vi "SimpleLiveApp.vi"() -> ()   [LabVIEW 2018]
uses:
  C:/Users/Public/Documents/Photometrics/PMQI-LabViewSamples/Examples/Dependencies/PVCamNET.dll
  Public/Documents/Photometrics/PMQI-LabViewSamples/Examples/Dependencies/PVCamNET.dll
panel:
  in  "Exposure Time":dbl
  in  "Live":bool
  in  "Camera Status":bool
  in  "Uninit":bool
  in  "Live stop":bool
  in  "Live start":bool
  in  "Init":bool
  # "SimpleLiveApp.vi\n\nDescription:\nThis sample code lets the user use live mode in an event driven structure.\n\nSteps to run:\n1. Click \"Run\"\n2. Click \"Open\"\n3. Enter Exposure Time\n4. Click \"Live start\"\n5. Click \"Live stop\"\n6. Click \"Close\""
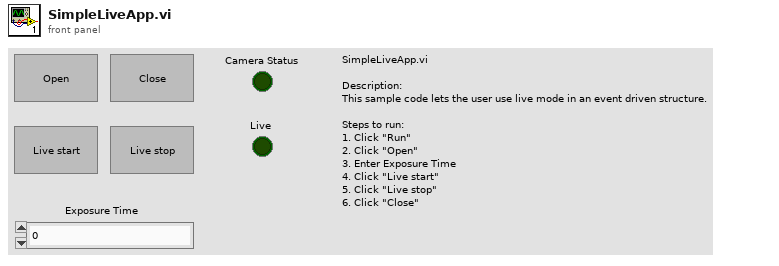
[diagram p1: front panel]
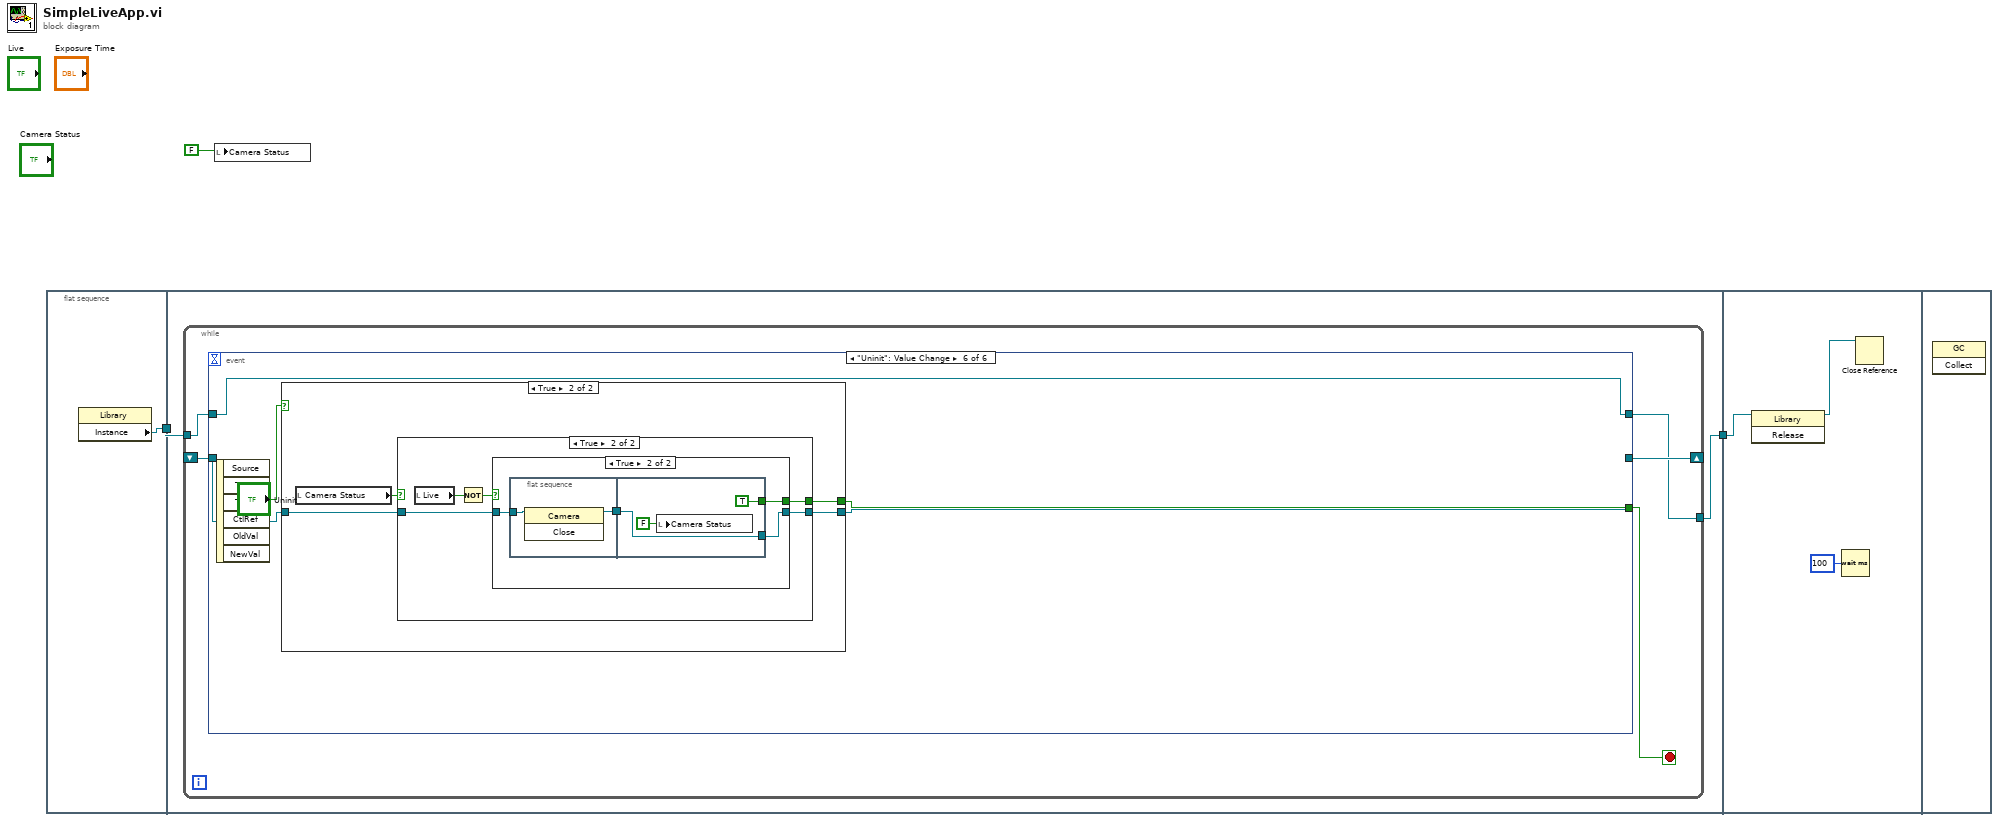
[diagram p0: block diagram]
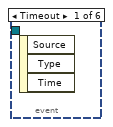
[diagram p2: hidden frame]
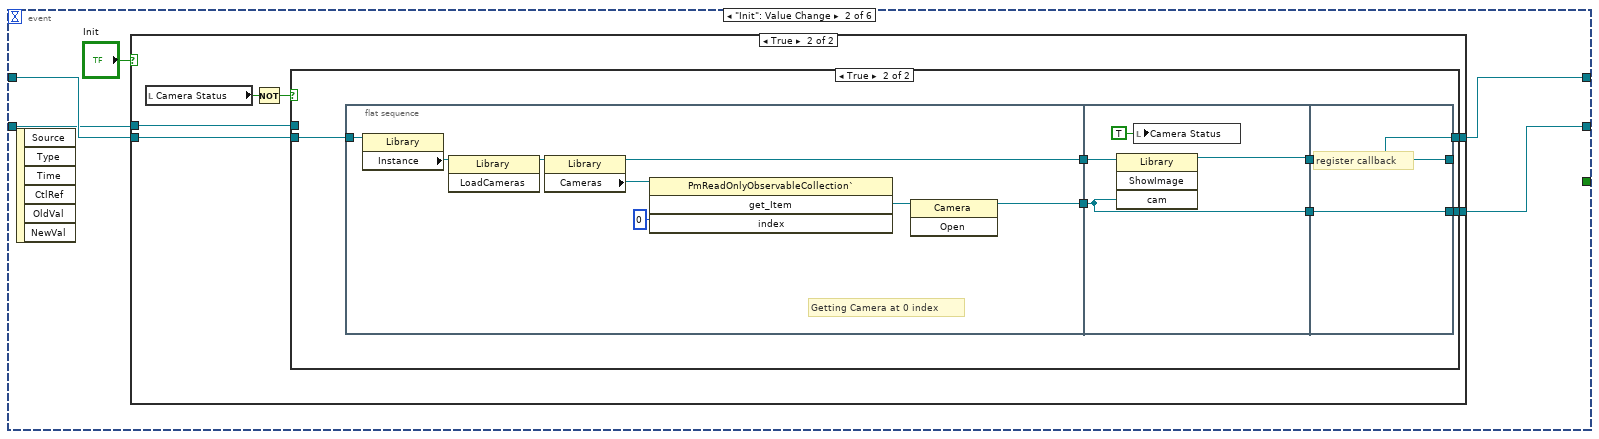
[diagram p3: hidden frame]
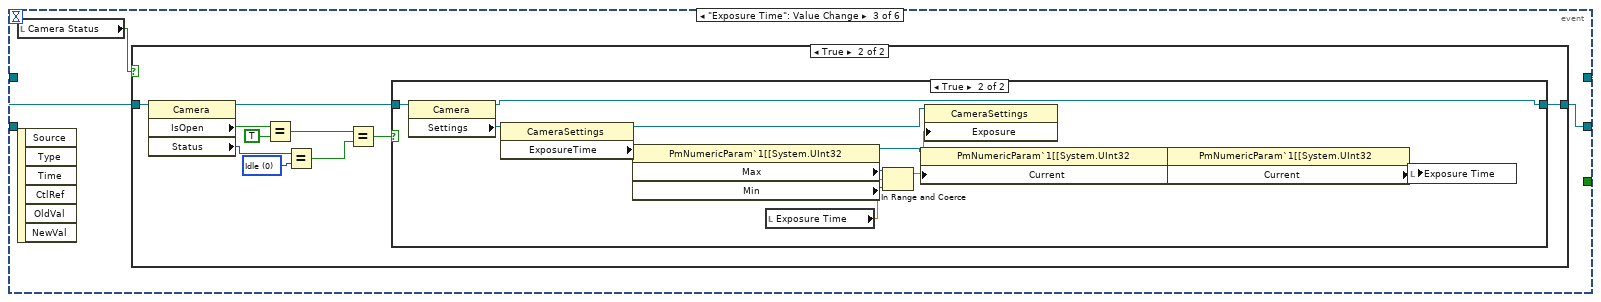
[diagram p6: hidden frame]
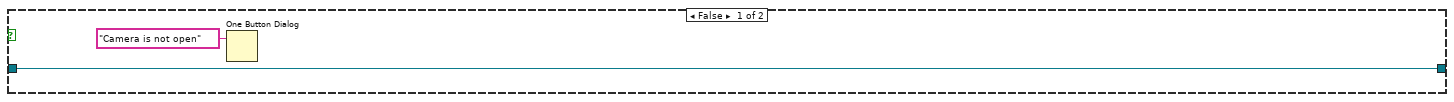
[diagram p7: hidden frame]
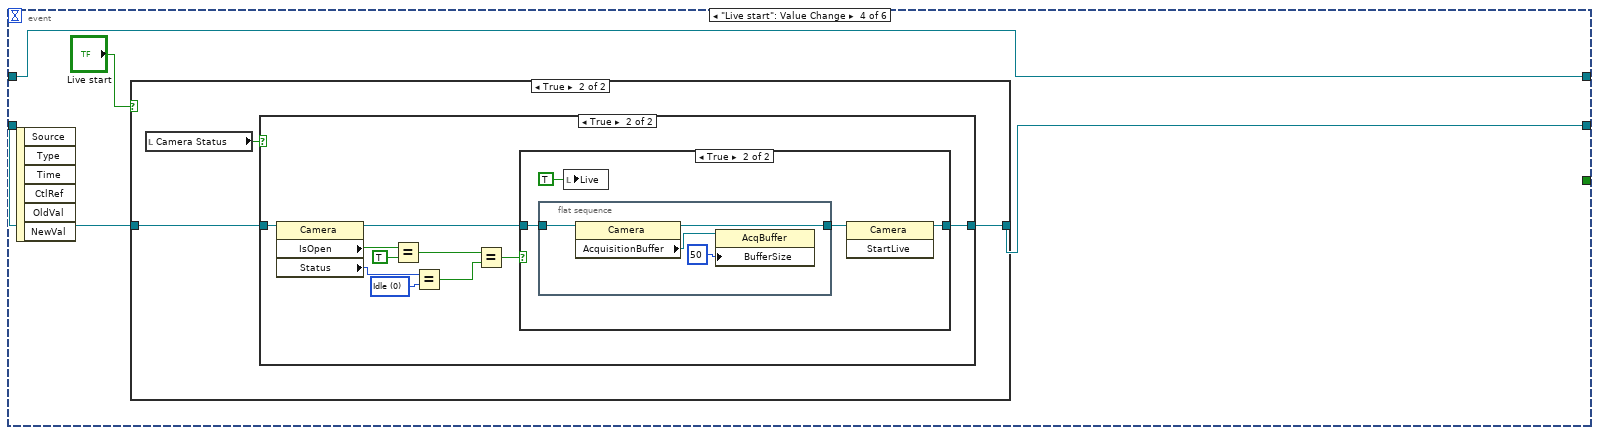
[diagram p9: hidden frame]
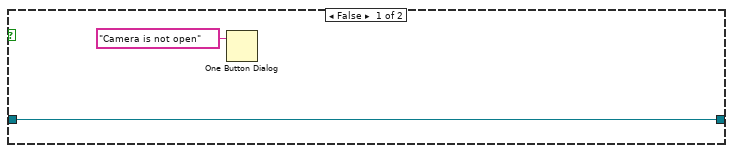
[diagram p11: hidden frame]
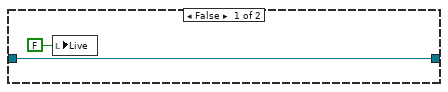
[diagram p12: hidden frame]
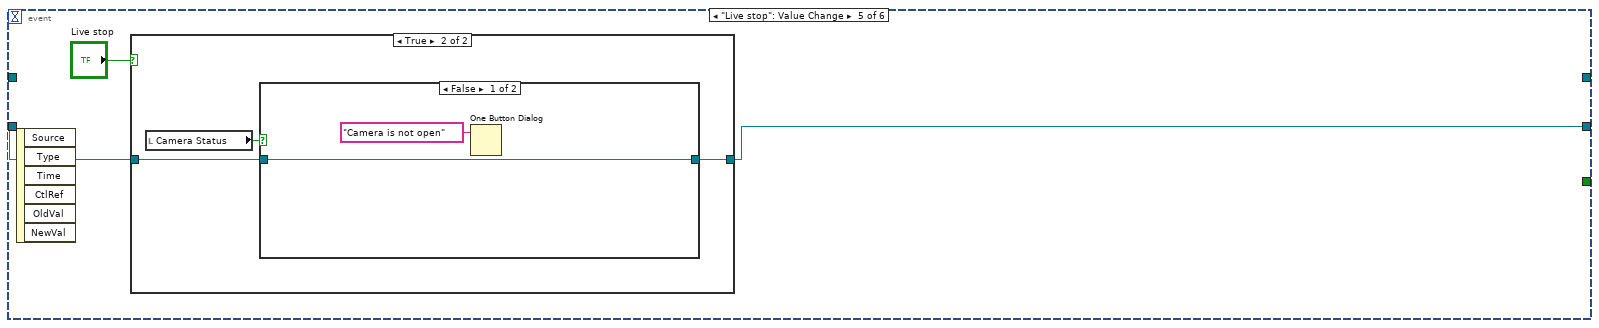
[diagram p13: hidden frame]
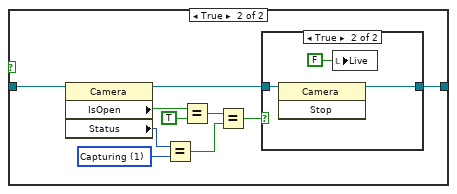
[diagram p15: hidden frame]
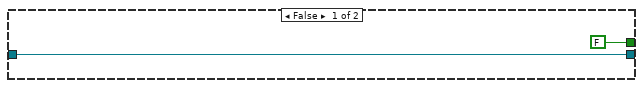
[diagram p17: hidden frame]
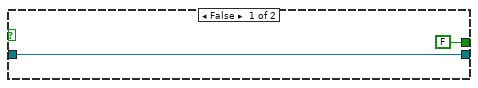
[diagram p18: hidden frame]
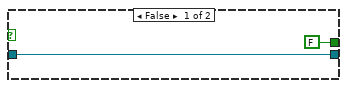
[diagram p19: hidden frame]
diagram:
  n1 = flat-sequence {
    tunnel: [w4] -> w3
    tunnel: w3 -> [w6]
    tunnel: [w5] -> w2
    tunnel: w2 -> [w160]
    frame #0 {
      n2 = property class="Library"() -> ("Instance"=w4:refnum<k24>)  [unwired: 2 in, 2 out]
    }
    frame #1 {
      n3 = while {
        tunnel: w6 -> [w11]
        shift-right: [w10] -> _
        shift-left: _ -> [w8]
        tunnel: [w9] -> w5
        stop <- w7 stop-if-true
        n4 = event shown="[5] \"Uninit\": Value Change" {
          selector: _ -> [_ _ _ _ _ _]
          dyn-events: _ -> [_ _ _ _ _ _]
          timeout: _ -> [_ _ _ _ _ _]
          tunnel: w11 -> [_ w16 w49 w77 _ w132]
          tunnel: [_ w15 w50 w78 w107 w133] -> w10
          tunnel: [_ w14 w49 w77 _ w132] -> w9
          tunnel: w8 -> [_ w13 w51 w79 w108 w134]
          tunnel: [_ _ _ _ _ w131] -> w7
          event Timeout {
            n5 = event-data() -> ()  [unwired: 1 in, 3 out]
          }
          event "Init": Value Change {
            n6 = event-data() -> ()  [unwired: 1 in, 6 out]
            n7 = case shown="True" "Init" {
              tunnel: w16 -> [w18 w24]
              tunnel: [w17 w23] -> w15
              tunnel: [w18 w22] -> w14
              tunnel: w13 -> [w17 w19]
              frame False {
              }
              frame True {
                n8 = local read "Camera Status"() -> (w21:bool)
                n9 = Not(x=w21) -> (.not. x?=w20:bool)
                n10 = case shown="True" w20 {
                  tunnel: w24 -> [w25 w31]
                  tunnel: [w26 w30] -> w23
                  tunnel: [w25 w29] -> w22
                  tunnel: w19 -> [w26 _]
                  frame False {
                  }
                  frame True {
                    n11 = flat-sequence {
                      tunnel: w31 -> [w36]
                      tunnel: [w38] -> w33
                      tunnel: [w37] -> w32
                      tunnel: w33 -> [w44]
                      tunnel: w32 -> [w45]
                      tunnel: [w45] -> w28
                      tunnel: [w43] -> w27
                      tunnel: [w46] -> w29
                      tunnel: [w47] -> w30
                      tunnel: w28 -> [w47]
                      tunnel: w27 -> [w46]
                      frame #0 {
                        # "Getting Camera at 0 index"
                        n12 = property class="Library"(reference=w36) -> ("Instance"=w35:refnum<k24>)  [unwired: 1 in, 2 out]
                        n13 = invoke class="Library" method="LoadCameras"(reference=w35) -> (reference out=w34:refnum<k24>)  [unwired: 2 in, 2 out]
                        n14 = property class="Library"(reference=w34) -> (reference out=w38:refnum<k24>, "Cameras"=w41:refnum<k24>)  [unwired: 1 in, 1 out]
                        n15 = invoke class="PmReadOnlyObservableCollection`" method="get_Item"(reference=w41, "index"=0) -> ("get_Item"=w39:refnum<k24>)  [unwired: 2 in, 3 out]
                        n16 = invoke class="Camera" method="Open"(reference=w39) -> (reference out=w37:refnum<k24>)  [unwired: 2 in, 2 out]
                      }
                      frame #1 {
                        n17 = invoke class="Library" method="ShowImage"(reference=w44, "cam"=w45) -> (reference out=w43:refnum<k24>)  [unwired: 2 in, 3 out]
                        n18 = local write "Camera Status"(TRUE ("Camera Status")) -> ()
                      }
                      frame #2 {
                        # "register callback"
                      }
                    }
                  }
                }
              }
            }
          }
          event "Exposure Time": Value Change {
            n19 = local read "Camera Status"() -> (w48:bool)
            n20 = event-data() -> ()  [unwired: 1 in, 6 out]
            n21 = case shown="True" w48 {
              tunnel: w51 -> [w53 w57]
              tunnel: [w53 w54] -> w50
              frame False {
                n22 = One Button Dialog(message="Camera is not open") -> ()  [unwired: 1 in, 1 out]
              }
              frame True {
                w62 = 0 items=["Idle", "Capturing"] ("Status")
                n23 = property class="Camera"(reference=w57) -> (reference out=w55:refnum<k24>, "IsOpen"=w61:bool, "Status"=w63:i32)  [unwired: 1 in, 1 out]
                n24 = Equal?(x=w61, y=TRUE) -> (x = y?=w59:bool)
                n25 = Equal?(x=w63, y=w62) -> (x = y?=w58:bool)
                n26 = Equal?(x=w59, y=w58) -> (x = y?=w56:bool)
                n27 = case shown="True" w56 {
                  tunnel: w55 -> [w64 w76]
                  tunnel: [w64 w65] -> w54
                  frame False {
                  }
                  frame True {
                    n28 = property class="Camera"(reference=w76) -> (reference out=w65:refnum<k24>, "Settings"=w75:refnum<k24>)  [unwired: 1 in, 1 out]
                    n29 = property class="CameraSettings"(reference=w75) -> (reference out=w68:refnum<k24>, "ExposureTime"=w69:refnum<k24>)  [unwired: 1 in, 1 out]
                    n30 = property class="PmNumericParam`1[[System.UInt32"(reference=w69) -> (reference out=w72:refnum<k24>, "Max"=w74:u32, "Min"=w73:u32)  [unwired: 1 in, 1 out]
                    n31 = local read "Exposure Time"() -> (w67:dbl)
                    n32 = In Range and Coerce(upper limit=w74, x=w67, lower limit=w73) -> (coerced(x)=w70:dbl)  [unwired: 1 out]
                    n33 = property class="PmNumericParam`1[[System.UInt32"(reference=w72, "Current"=w70) -> (reference out=w71:refnum<k24>)  [unwired: 1 in, 1 out]
                    n34 = property class="CameraSettings"(reference=w68, "Exposure"=w70) -> ()  [unwired: 1 in, 2 out]
                    n35 = property class="PmNumericParam`1[[System.UInt32"(reference=w71) -> ("Current"=w66:u32)  [unwired: 1 in, 2 out]
                    n36 = local write "Exposure Time"(w66) -> ()
                  }
                }
              }
            }
          }
          event "Live start": Value Change {
            n37 = event-data() -> ()  [unwired: 1 in, 6 out]
            n38 = case shown="True" "Live start" {
              tunnel: w79 -> [w81 w84]
              tunnel: [w81 w83] -> w78
              frame False {
              }
              frame True {
                n39 = local read "Camera Status"() -> (w82:bool)
                n40 = case shown="True" w82 {
                  tunnel: w84 -> [w85 w90]
                  tunnel: [w85 w88] -> w83
                  frame False {
                    n41 = One Button Dialog(message="Camera is not open") -> ()  [unwired: 1 in, 1 out]
                  }
                  frame True {
                    w95 = 0 items=["Idle", "Capturing"] ("Status")
                    n42 = property class="Camera"(reference=w90) -> (reference out=w89:refnum<k24>, "IsOpen"=w94:bool, "Status"=w96:i32)  [unwired: 1 in, 1 out]
                    n43 = Equal?(x=w94, y=TRUE) -> (x = y?=w92:bool)
                    n44 = Equal?(x=w96, y=w95) -> (x = y?=w91:bool)
                    n45 = Equal?(x=w92, y=w91) -> (x = y?=w87:bool)
                    n46 = case shown="True" w87 {
                      tunnel: w89 -> [w98 w100]
                      tunnel: [w98 w101] -> w88
                      frame False {
                        n47 = local write "Live"(FALSE ("Live 2")) -> ()
                      }
                      frame True {
                        n48 = flat-sequence {
                          tunnel: w100 -> [w106]
                          tunnel: [w103] -> w99
                          frame #0 {
                            n49 = property class="Camera"(reference=w106) -> (reference out=w103:refnum<k24>, "AcquisitionBuffer"=w105:refnum<k24>)  [unwired: 1 in, 1 out]
                            n50 = property class="AcqBuffer"(reference=w105, "BufferSize"=50) -> ()  [unwired: 1 in, 2 out]
                          }
                        }
                        n51 = local write "Live"(TRUE ("Live")) -> ()
                        n52 = invoke class="Camera" method="StartLive"(reference=w99) -> (reference out=w101:refnum<k24>)  [unwired: 2 in, 2 out]
                      }
                    }
                  }
                }
              }
            }
          }
          event "Live stop": Value Change {
            n53 = event-data() -> ()  [unwired: 1 in, 6 out]
            n54 = case shown="True" "Live stop" {
              tunnel: w108 -> [w110 w113]
              tunnel: [w110 w112] -> w107
              frame False {
              }
              frame True {
                n55 = local read "Camera Status"() -> (w111:bool)
                n56 = case shown="False" w111 {
                  tunnel: w113 -> [w115 w125]
                  tunnel: [w115 w122] -> w112
                  frame False {
                    n57 = One Button Dialog(message="Camera is not open") -> ()  [unwired: 1 in, 1 out]
                  }
                  frame True {
                    w120 = 1 items=["Idle", "Capturing"] ("Status")
                    n58 = property class="Camera"(reference=w125) -> (reference out=w123:refnum<k24>, "IsOpen"=w119:bool, "Status"=w121:i32)  [unwired: 1 in, 1 out]
                    n59 = Equal?(x=w121, y=w120) -> (x = y?=w116:bool)
                    n60 = Equal?(x=w119, y=TRUE) -> (x = y?=w117:bool)
                    n61 = Equal?(x=w117, y=w116) -> (x = y?=w124:bool)
                    n62 = case shown="True" w124 {
                      tunnel: w123 -> [w126 w129]
                      tunnel: [w126 w128] -> w122
                      frame False {
                      }
                      frame True {
                        n63 = invoke class="Camera" method="Stop"(reference=w129) -> (reference out=w128:refnum<k24>)  [unwired: 2 in, 2 out]
                        n64 = local write "Live"(FALSE ("Live 2")) -> ()
                      }
                    }
                  }
                }
              }
            }
          }
          event "Uninit": Value Change {
            n65 = event-data() -> ()  [unwired: 1 in, 6 out]
            n66 = case shown="True" "Uninit" {
              tunnel: w134 -> [w136 w140]
              tunnel: [w136 w139] -> w133
              tunnel: [FALSE ("Camera Status") w137] -> w131
              frame False {
              }
              frame True {
                n67 = local read "Camera Status"() -> (w138:bool)
                n68 = case shown="True" w138 {
                  tunnel: w140 -> [w142 w147]
                  tunnel: [w142 w146] -> w139
                  tunnel: [FALSE ("Camera Status") w145] -> w137
                  frame False {
                  }
                  frame True {
                    n69 = local read "Live"() -> (w143:bool)
                    n70 = Not(x=w143) -> (.not. x?=w144:bool)
                    n71 = case shown="True" w144 {
                      tunnel: w147 -> [w149 w152]
                      tunnel: [w149 w151] -> w146
                      tunnel: [FALSE ("Camera Status") w150] -> w145
                      frame False {
                      }
                      frame True {
                        n72 = flat-sequence {
                          tunnel: w152 -> [w155]
                          tunnel: [w154] -> w153
                          tunnel: [w158] -> w151
                          tunnel: w153 -> [w158]
                          tunnel: [TRUE ("Camera Status")] -> w150
                          frame #0 {
                            n73 = invoke class="Camera" method="Close"(reference=w155) -> (reference out=w154:refnum<k24>)  [unwired: 2 in, 2 out]
                          }
                          frame #1 {
                            n74 = local write "Camera Status"(FALSE ("Camera Status")) -> ()
                          }
                        }
                      }
                    }
                  }
                }
              }
            }
          }
        }
      }
    }
    frame #2 {
      n75 = invoke class="Library" method="Release"(reference=w160) -> (reference out=w161:refnum<k24>)  [unwired: 2 in, 2 out]
      n76 = Wait (ms)(milliseconds to wait=u32 100) -> ()  [unwired: 1 out]
      n77 = Close Reference(reference=w161) -> ()  [unwired: 1 in, 1 out]
    }
    frame #3 {
      n78 = invoke class="GC" method="Collect"() -> ()  [unwired: 3 in, 3 out]
    }
  }
  n79 = local write "Camera Status"(FALSE ("Camera Status")) -> ()
